vi "solar_voy_def Export (Packet).vi"(10 "HDR_ID_NAME ('HDR_ID')":string="HDR_ID", 11 "PACKET":T2 {"last_time" format="%<%H:%M:%S%3u %m/%d/%y>T"}) -> (0 "ITEM VALUES (ASCII)":string[](array[string]), 1 "ITEM TYPES":T1[](array[typedef]), 2 "ITEM DEFS":string[](array[string]), 3 "PACKET Definition":string)   [LabVIEW 2018]
doc: "This exports a COSMOS definition packet to string."
uses:
  solar_voy_def_ctl ITEM.ctl
  solar_voy_def_ctl PACKET.ctl
  solar_voy_def_ctl ITEM TYPE.ctl
  type/solar_type Item Type.ctl
  solar_voy_def_ctl PACKET_ID.ctl
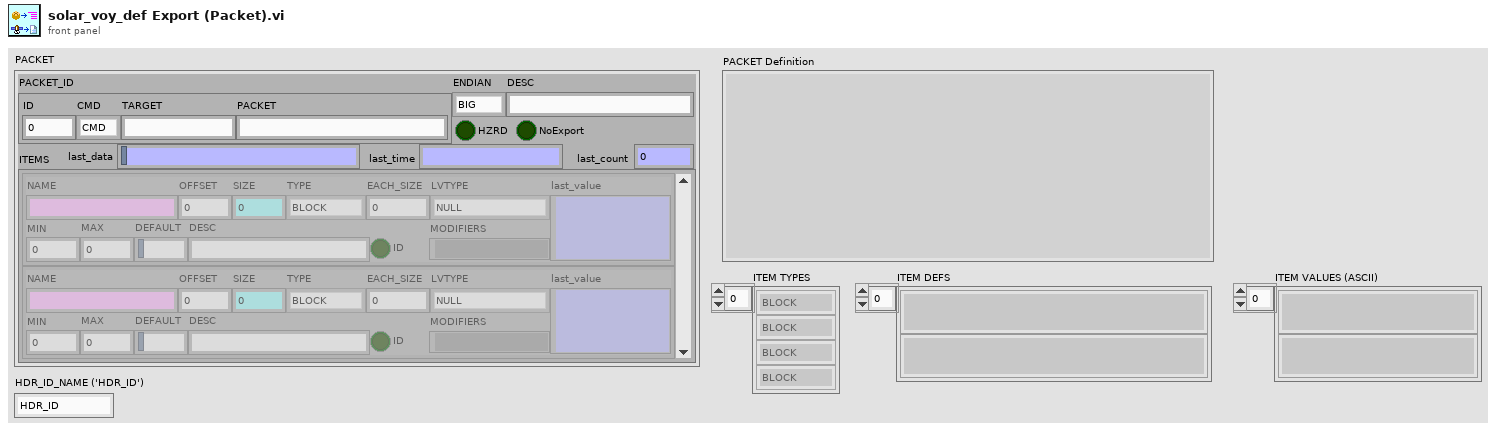
[diagram p1: front panel]
types:
  T1 = typedef "solar_voy_def_ctl ITEM TYPE.ctl" = enum8{"BLOCK", "INT", "UINT", "FLOAT", "STRING"}
  T2 = typedef "solar_voy_def_ctl PACKET.ctl" = cluster{"PACKET_ID":T3, "ENDIAN":enum8{"BIG", "LITTLE"}, "DESC":string, "HZRD":bool, "ITEMS":T4[], "NoExport":bool, "last_time":timestamp, "last_count":u32, "last_data":string}
  T3 = typedef "solar_voy_def_ctl PACKET_ID.ctl" = cluster{"ID":u16, "CMD":enum8{"CMD", "TLM"}, "TARGET":string, "PACKET":string}
  T4 = typedef "solar_voy_def_ctl ITEM.ctl" = cluster{"NAME":string, "OFFSET":i32, "SIZE":i32, "TYPE":T1, "EACH_SIZE":i32, "LVTYPE":T5, "MIN":dbl, "MAX":dbl, "DEFAULT":string, "DESC":string, "ID":bool, "MODIFIERS":variant, "last_value":variant}
  T5 = typedef "solar_type Item Type.ctl" = enum16{"NULL", "UNKNOWN", "CLUSTER", "I8", "I16", "I32", "I64", "U8", "U16", "U32", "U64", "U8_ENUM", "U16_ENUM", "U32_ENUM", "SGL", "DBL", "BOOLEAN", "STRING", "PATH", "VISA", "TAG", "TIME", "I8_1D", "I16_1D", "I32_1D", "I64_1D", "U8_1D", "U16_1D", "U32_1D", "U64_1D", "U8_ENUM_1D", "U16_ENUM_1D", "U32_ENUM_1D", "SGL_1D", "DBL_1D", "BOOLEAN_1D", "STRING_1D", "PATH_1D", "VISA_1D", "TAG_1D", "TIME_1D", "I8_2D", "I16_2D", "I32_2D", "I64_2D", "U8_2D", "U16_2D", "U32_2D", "U64_2D", "U8_ENUM_2D", "U16_ENUM_2D", "U32_ENUM_2D", "SGL_2D", "DBL_2D", "BOOLEAN_2D", "STRING_2D", "PATH_2D", "VISA_2D", "TAG_2D", "TIME_2D"}
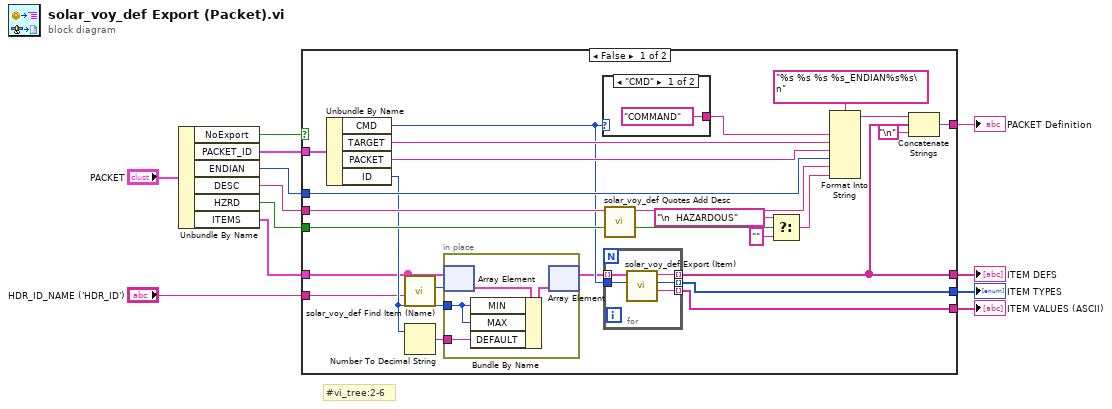
[diagram p0: block diagram]
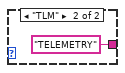
[diagram p2: hidden frame]
diagram:
  # "#vi_tree:2-6"
  n1 = Unbundle By Name("PACKET") -> ("NoExport"=w5:bool, "PACKET_ID"=w8:T3, "ENDIAN"=w11:enum8{"BIG", "LITTLE"}, "DESC"=w7:string, "HZRD"=w10:bool, "ITEMS"=w6:T4[])
  n2 = case shown="False" w5 {
    tunnel: w11 -> [w37 _]
    tunnel: w10 -> [w36 _]
    tunnel: [w30 _] -> w9
    tunnel: w8 -> [w23 _]
    tunnel: w7 -> [w28 _]
    tunnel: w6 -> [w16 _]
    tunnel: [w25 _] -> w4
    tunnel: [w24 _] -> w3
    tunnel: "HDR_ID_NAME ('HDR_ID')" -> [w15 _]
    tunnel: [w13 _] -> w1
    frame False {
      n3 = Unbundle By Name(w23) -> ("CMD"=w20:enum8{"CMD", "TLM"}, "TARGET"=w22:string, "PACKET"=w21:string, "ID"=w17:u16)
      n4 = call "solar_voy_def Find Item (Name).vi"("ITEM_NAME"=w15, "ITEMS"=w16) -> ("Index"=w14:i32)  [unwired: 9 in]
      n5 = Number To Decimal String(number=w17) -> (decimal integer string=w19:string)  [unwired: 1 in]
      n6 = in-place {
        in-place-border: w17 -> [w39]
        in-place-border: w19 -> [w38]
        n7 = in-place-array #1(w16, w14) -> (w41:T4)
        n8 = Bundle By Name(cluster=w41, "MIN"=w39, "MAX"=w39, "DEFAULT"=w38) -> (w40:T4)
        n9 = in-place-array #1(w40) -> (w18:T4[])  [unwired: 1 out]
      }
      n10 = case shown="\"CMD\"" w20 {
        tunnel: ["COMMAND" "TELEMETRY"] -> w29
        frame "CMD" {
        }
        frame "TLM" {
        }
      }
      n11 = for {
        tunnel: w18 -> [w48] mode=indexing
        tunnel: [w47] -> w25 mode=indexing
        tunnel: w20 -> [w46]
        tunnel: [w45] -> w24 mode=indexing
        tunnel: [w44] -> w13 mode=indexing
        n12 = call "solar_voy_def Export (Item).vi"("CMD"=w46, "ITEM"=w48) -> ("Last Value (ASCII)"=w44:string, "TYPE"=w45:T1, "ITEM_DEF"=w47:string)  [unwired: 7 in]
      }
      n13 = call "solar_voy_def Quotes Add Desc.vi"("Description"=w28) -> ("Description with Comments"=w27:string)  [unwired: 10 in]
      n14 = Select(t="\n  HAZARDOUS", s=w36, f="") -> (s? t:f=w33:string)
      n15 = Format Into String(format string="%s %s %s %s_ENDIAN%s%s\n", w29, w22, w21, w37, w27, w33) -> (resulting string=w31:string)  [unwired: 2 in, 1 out]
      n16 = Concatenate Strings(w31, w25, "\n" ("Line Feed Constant")) -> (w30:string)
    }
    frame True {
      # "No Export\n- Do not export packet"
    }
  }
  "PACKET Definition" <- w9
  "ITEM DEFS" <- w4
  "ITEM TYPES" <- w3
  "ITEM VALUES (ASCII)" <- w1
